vi "IsActive.vi"(8 "error in":errorcluster, 11 "Attribute in":refnum<class "Attribute.lvclass">) -> (0 "error out":errorcluster, 2 "IsActive":bool, 3 "Attribute out":refnum<class "Attribute.lvclass">)   [LabVIEW 2021, in "ProligentXMLGenerator.lvlib" / "Attribute.lvclass"]
uses:
  Attribute.lvclass
  Attribute.lvclass/Attribute.ctl
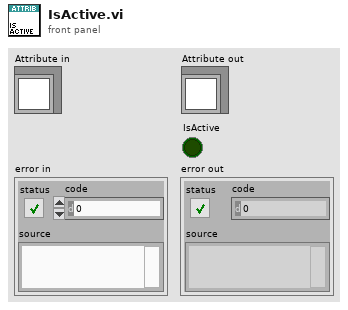
[diagram p1: front panel]
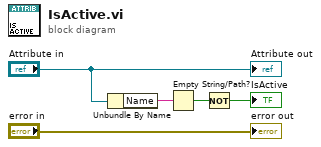
[diagram p0: block diagram]
diagram:
  n1 = Unbundle By Name("Attribute in") -> ("Name"=w3:string)
  n2 = Empty String/Path?(string/path=w3) -> (empty?=w2:bool)
  n3 = Not(x=w2) -> (.not. x?=→"IsActive":bool)
  "error out" <- "error in"
  "Attribute out" <- "Attribute in"
